vi "SetFrequencyControl.vi"(0 "Frequency Control Cluster":T1={"Actual Value"=-2147483648, "Setpoint [a.u.]"=-inf, "Min"=-inf, "Invert Polarity"=-2147483648, "Max"=-inf, "df"=-inf, "P"=-inf, "f excite"=-inf, "I"=-inf, "state"=FALSE} {"I" format="%#_g mHz"; "f excite" format="%#_g kHz"; "df" format="%#_g kHz"; "Max" format="%#_g kHz"; "Invert Polarity" items=["[read only]"=-2147483648, "No"=0, "Yes"=1]; "Min" format="%#_g kHz"; "Actual Value" items=["[read only]"=-2147483648, "ADC 1"=0, "ADC 2"=1, "ADC 3"=2, "ADC 4"=3, "ADC 5"=4, "ADC 6"=5, "HF 1 df"=8, "HF 1 Ampl"=13, "HF 1 Phase"=14, "LockIn Ampl"=16, "LockIn Phase"=17, "Counter"=23]}, 5 "error in":T4) -> (14 "Output Cluster":T1={"Actual Value"=-214748348, "Setpoint [a.u.]"=-inf, "Min"=-inf, "Invert Polarity"=-2147483648, "Max"=-inf, "df"=-inf, "P"=-2147483600.0, "f excite"=-inf, "I"=-inf, "state"=FALSE} {"I" format="%#_g mHz"; "f excite" format="%#_g kHz"; "df" format="%#_g kHz"; "Max" format="%#_g kHz"; "Invert Polarity" items=["[read only]"=-2147483648, "No"=0, "Yes"=1]; "Min" format="%#_g kHz"; "Actual Value" items=["[read only]"=-2147483648, "ADC 1"=0, "ADC 2"=1, "ADC 3"=2, "ADC 4"=3, "ADC 5"=4, "ADC 6"=5, "HF 1 df"=8, "HF 1 Ampl"=13, "HF 1 Phase"=14, "LockIn Ampl"=16, "LockIn Phase"=17, "Counter"=23]}, 19 "error out":T4)   [LabVIEW 2016]
doc: "This VI sets up all parameters concerning the frequency control. The input cluster contains the following items:\n\n- Actual Value (integer) [0-5 -- ADC1-6; 8 -- AFM df; 13 -- AFM df; 13 -- AFM Aosc; 14 -- AFM Phase; 16 -- LockIn Ampl; 17 -- LockIn Phase]\n- Min in kHz (float) [0 to 500]\n- Max in kHz (float) [0 to 500]\n- P (float) [0 to 1]\n- I in uHz (float) [0 to 1000000000]\n- Setpoint; Unit depends on the input \"Actual Value\": mV, Hz or degree (float) [without restraint]\n- Invert Polarity (integer) [0 -- no; 1 -- yes]\n- df in kHz (float) [without restraint]\n- f excite in kHz (float) [0 to 2000]\nBy passing -Inf (float) or -2147483648 (integer) as input values, the corresponding parameter(s) will be read out."
uses:
  Controls/Frequency-Control_Parameters.ctl
  Controls/Actual-Value_Selection.ctl
  Controls/Invert-Polarity_Selection.ctl
  Controls/Error_Out.ctl
  Files_ASC500/DLL/ASC500_RemoteControlV27.dll
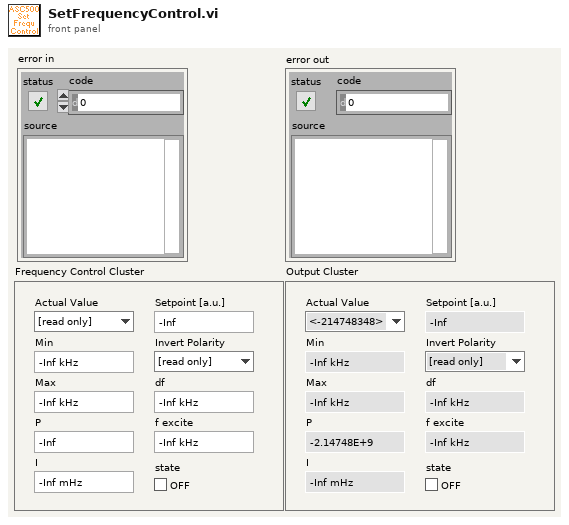
[diagram p1: front panel]
types:
  T1 = typedef "Frequency-Control_Parameters.ctl" = cluster{"Actual Value":T2, "Setpoint [a.u.]":sgl, "Min":sgl, "Invert Polarity":T3, "Max":sgl, "df":sgl, "P":sgl, "f excite":sgl, "I":sgl, "state":bool}
  T2 = typedef "Actual-Value_Selection.ctl" = i32
  T3 = typedef "Invert-Polarity_Selection.ctl" = i32
  T4 = typedef "Error_Out.ctl" = errorcluster
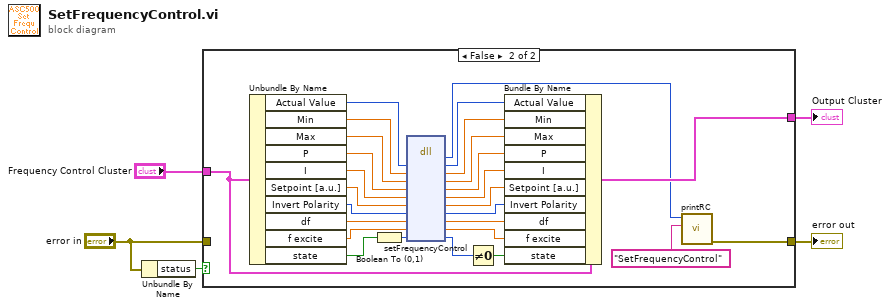
[diagram p0: block diagram]
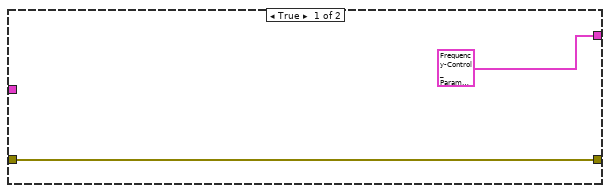
[diagram p2: hidden frame]
diagram:
  n1 = Unbundle By Name("error in") -> ("status"=w5:bool)
  n2 = case shown="False" w5 {
    tunnel: [w6 w14] -> w1
    tunnel: "Frequency Control Cluster" -> [_ w18]
    tunnel: [T1 {"Actual Value"=-2147483648, "Setpoint [a.u.]"=-inf, "Min"=-inf, "Invert Polarity"=-2147483648, "Max"=-inf, "df"=-inf, "P"=-2147483600.0, "f excite"=-inf, "I"=-inf, "state"=FALSE} ("Frequency Control Cluster") w17] -> w3
    tunnel: "error in" -> [w6 _]
    frame True {
    }
    frame False {
      n3 = Unbundle By Name(w18) -> ("Actual Value"=w34:T2, "Min"=w33:sgl, "Max"=w32:sgl, "P"=w31:sgl, "I"=w30:sgl, "Setpoint [a.u.]"=w29:sgl, "Invert Polarity"=w28:T3, "df"=w15:sgl, "f excite"=w20:sgl, "state"=w10:bool)
      n4 = Boolean To (0,1)(Boolean=w10) -> (0, 1=w11:i16)
      n5 = dll-call lib="G:/SCMOperations/Share/ELE/Produkt Information/ASC500/04 Remote Control/02 development versions/2018Nov06/Files_ASC500/DLL/ASC500_RemoteControlV27.dll" fn="setFrequencyControl"("Actual Value"=w34, "Min"=w33, "Max"=w32, "P"=w31, "I"=w30, "Setpoint"=w29, "Invert Polarity"=w28, "df"=w15, "f excite"=w20, "state"=w11) -> ("return type"=w13:i32, "Actual Value"=w27:i32, "Min"=w26:sgl, "Max"=w25:sgl, "P"=w24:sgl, "I"=w23:sgl, "Setpoint"=w22:sgl, "Invert Polarity"=w21:i32, "df"=w16:sgl, "f excite"=w19:sgl, "state"=w8:i32)  [unwired: 3 in, 2 out]
      n6 = Not Equal To 0?(x=w8) -> (x != 0?=w9:bool)
      n7 = Bundle By Name(cluster=w18, "Actual Value"=w27, "Min"=w26, "Max"=w25, "P"=w24, "I"=w23, "Setpoint [a.u.]"=w22, "Invert Polarity"=w21, "df"=w16, "f excite"=w19, "state"=w9) -> (w17:T1)
      n8 = call "printRC.vi"("additional information"="SetFrequencyControl", "RC"=w13) -> ("error out"=w14:T4)  [unwired: 9 in]
    }
  }
  "error out" <- w1
  "Output Cluster" <- w3
